vi "HSV Distance Comparison.vi"(10 "Image 2":path, 11 "Image 1":path) -> (3 "HSV Distance":dbl)   [LabVIEW 2015, in "HSV Distance Comparison.lvclass"]
uses:
  HSV Distance Comparison.lvclass
  Image Comparison/Image Comparison.lvclass
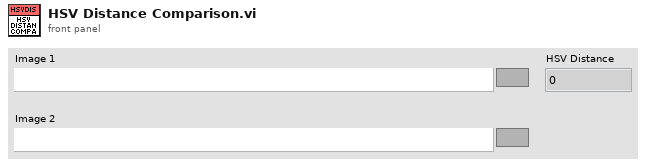
[diagram p1: front panel]
types:
  T1 = typedef "imagedata.ctl" = cluster{"image type":i32, "image depth":i32, "image":u8[], "mask":u8[], "colors":u32[], "Rectangle":cluster{"left":i16, "top":i16, "right":i16, "bottom":i16}}
  T2 = cluster{"H (deg)":dbl, "S (%)":dbl, "V (%)":dbl}[]
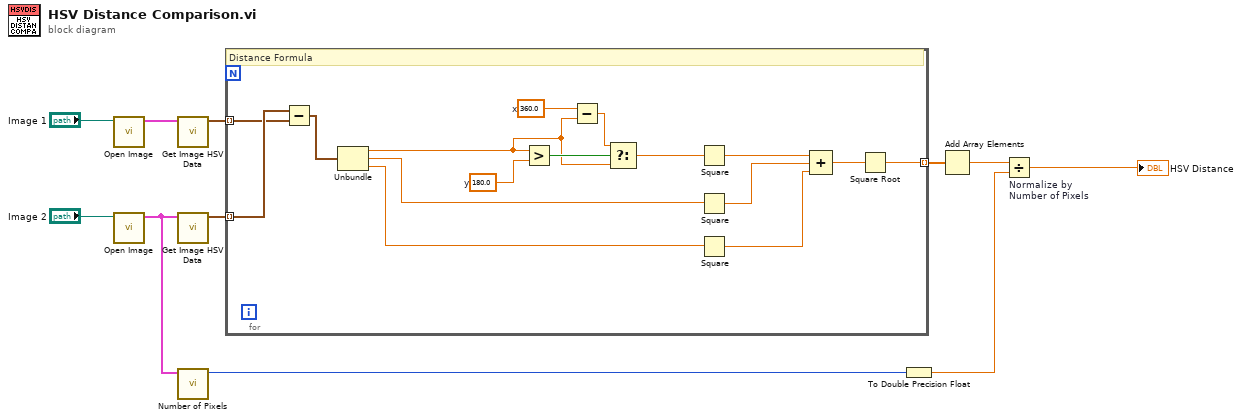
[diagram p0: block diagram]
diagram:
  n1 = call "Open Image.vi"("Image"="Image 1") -> ("image data"=w6:T1)  [unwired: 9 in, 1 out]
  n2 = call "Open Image.vi"("Image"="Image 2") -> ("image data"=w4:T1)  [unwired: 9 in, 1 out]
  n3 = call "Get Image HSV Data.vi"("image data"=w6) -> ("HSV[]"=w11:T2)  [unwired: 10 in]
  n4 = call "Get Image HSV Data.vi"("image data"=w4) -> ("HSV[]"=w10:T2)  [unwired: 10 in]
  n5 = call "Number of Pixels.vi"("image data"=w4) -> ("Number of Pixels"=w3:u64)  [unwired: 10 in]
  n6 = for {
    tunnel: w10 -> [w17] mode=indexing
    tunnel: w11 -> [w16] mode=indexing
    tunnel: [w25] -> w9 mode=indexing
    w22 = 360.0  # x
    w24 = 180.0  # y
    # "Distance Formula"
    n7 = Subtract(x=w17, y=w16) -> (x-y=w15:cluster{"H (deg)":dbl, "S (%)":dbl, "V (%)":dbl})
    n8 = Unbundle(w15) -> ("H (deg)"=w14:dbl, "S (%)"=w13:dbl, "V (%)"=w12:dbl)
    n9 = Greater?(x=w14, y=w24) -> (0:w23:bool)
    n10 = Subtract(x=w22, y=w14) -> (x-y=w21:dbl)
    n11 = Select(t=w21, s=w23, f=w14) -> (s? t:f=w20:dbl)
    n12 = Square(x=w20) -> (x^2=w19:dbl)
    n13 = Square(x=w13) -> (x^2=w27:dbl)
    n14 = Square(x=w12) -> (x^2=w18:dbl)
    n15 = Compound Arithmetic op=ADD(w19, w27, w18) -> (w26:dbl)
    n16 = Square Root(x=w26) -> (sqrt(x)=w25:dbl)
  }
  n17 = To Double Precision Float(number=w3) -> (double precision float=w1:dbl)
  n18 = Add Array Elements(numeric array=w9) -> (sum=w8:dbl)
  n19 = Divide "Normalize by\nNumber of Pixels"(x=w8, y=w1) -> (x/y=→"HSV Distance":dbl)
